vi "Send Send Task Outputs.vi"(4 "Status":string="Built", 6 "Build Specification Version":T1, 7 "Priority":T2=enum."Normal" caption="Message Priority (Normal)", 8 "error in (no error)":errorcluster, 9 "Generated files":path[](array[path]), 10 "Task":refnum<class "Task.lvclass">, 11 "Message Enqueuer in":refnum<class "Message Enqueuer.lvclass">) -> (0 "error out":errorcluster, 3 "Message Enqueuer out":refnum<class "Message Enqueuer.lvclass">)   [LabVIEW 2017, in "BuildWorker.lvlib" / "Send Task Outputs Msg.lvclass"]
doc: "Sends the <b>BuildWorker.lvlib:Send Task Outputs Msg.lvclass</b> message.\n\nThis message will call <b>Send Task Outputs.vi</b> on the <b>BuildWorker.lvlib:BuildWorker.lvclass</b> actor.\n\n<b>Send Task Outputs.vi Description</b>"
uses:
  Send Task Outputs Msg.lvclass
  <vilib>/ActorFramework/Message Enqueuer/Message Enqueuer.lvclass
  <vilib>/ActorFramework/Message Enqueuer/Message Priority.ctl
  Classes/Task Interface/Task/Task.lvclass
  <vilib>/AppBuilder/AB_API_Simple/Build Specification Version.ctl
  C:/Program Files (x86)/National Instruments/LabVIEW 2017/vi.lib/ActorFramework/Message/Message.lvclass
  Send Task Outputs Msg.lvclass/Send Task Outputs Msg.ctl
  <vilib>/ActorFramework/Message Enqueuer/Message Enqueuer.lvclass/Message Enqueuer.ctl
  <vilib>/ActorFramework/Message Priority Queue/Priority Enqueue.vi
  <vilib>/AppBuilder/AB_API_Simple/NI_App_Builder_API.lvlib
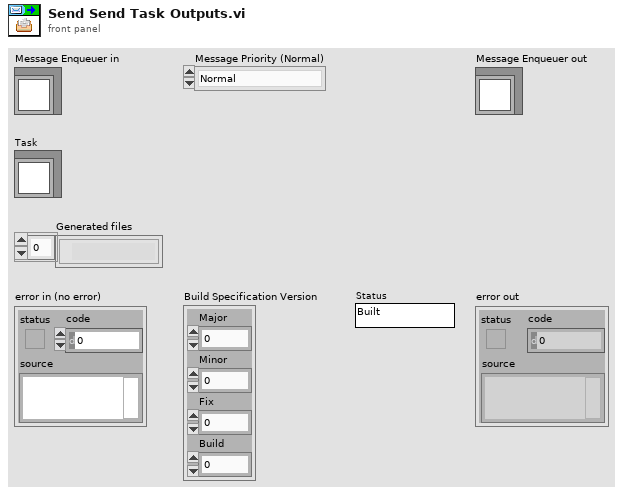
[diagram p1: front panel]
types:
  T1 = typedef "NI_App_Builder_API.lvlib/Build Specification Version.ctl" = cluster{"Major":u16, "Minor":u16, "Fix":u16, "Build":u16}
  T2 = typedef "Actor Framework.lvlib/Message Enqueuer.lvclass/Message Priority.ctl" = enum16{"Low", "Normal", "High"}
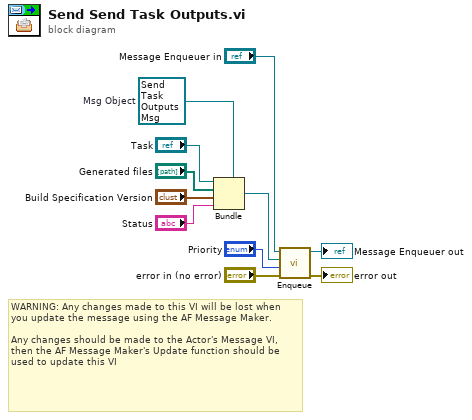
[diagram p0: block diagram]
diagram:
  w7 = refnum<class "Send Task Outputs Msg.lvclass"> refnum  # Msg Object
  # "WARNING: Any changes made to this VI will be lost when you update the message using the AF Message Maker.\n\nAny changes should be made to the Actor's Message VI, then the AF Message Maker's Update function should be used to update this VI"
  n1 = Bundle(cluster=w7, "Task", "Generated files", "Build Specification Version", "Status") -> (w2:refnum<class "Send Task Outputs Msg.lvclass">)
  n2 = call <vilib>:"Enqueue.vi"("error in (no error)"="error in (no error)", "Message Priority (Normal)"="Priority", "Message"=w2, "Message Enqueuer in"="Message Enqueuer in") -> ("error out"=→"error out":errorcluster, "Message Enqueuer out"=→"Message Enqueuer out":refnum<class "Message Enqueuer.lvclass">)  [unwired: 6 in]
